vi "JSON to LVObject - Base Class - Returns Matching Type.vi"() -> ()   [LabVIEW 2017, in "Tests.lvlib" / "Type Name Handling.lvlib"]
uses:
  Weather Forecast/Weather Forecast.lvclass
  Flatten To JSON Object/Flatten To JSON Object.lvclass
  Flatten To JSON Object/Type Name Handling.ctl
  Flatten To JSON Object/Flatten To JSON Object.lvclass/Flatten To JSON Object.ctl
  Flatten To JSON Object/Write Type Name Handling.vi
  <vilib>/addons/_JKI Toolkits/Caraya/classes/Assert/Assert Equal Value and Type_Variant.vi
  Type Name Handling.lvlib
  <vilib>/addons/_JKI Toolkits/Caraya/classes/Test/Test.lvclass
  <vilib>/addons/_JKI Toolkits/Caraya/classes/Assert/Assert.lvclass
panel:
  out "error out":errorcluster
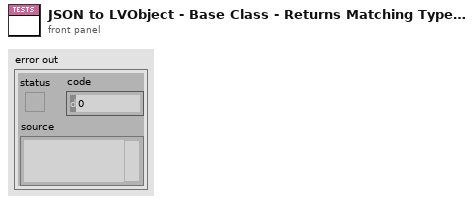
[diagram p1: front panel]
types:
  T1 = typedef "Flatten To JSON Object.lvclass/Type Name Handling.ctl" = enum16{"None", "Inline"}
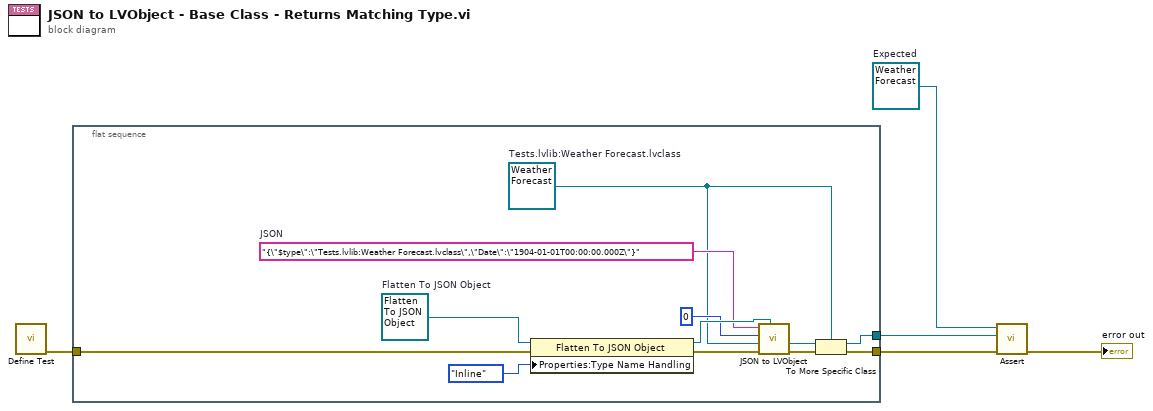
[diagram p0: block diagram]
diagram:
  w1 = refnum<class "Weather Forecast.lvclass"> refnum  # Expected
  n1 = call <vilib>:"Define Test.vi"() -> ("error out"=w5:errorcluster)  [unwired: 11 in]
  n2 = flat-sequence {
    tunnel: w5 -> [w15]
    tunnel: [w7] -> w4
    tunnel: [w9] -> w3
    frame #0 {
      w12 = "{\"$type\":\"Tests.lvlib:Weather Forecast.lvclass\",\"Date\":\"1904-01-01T00:00:00.000Z\"}"  # JSON
      w17 = refnum<class "Flatten To JSON Object.lvclass"> refnum  # Flatten To JSON Object
      w6 = refnum<class "Weather Forecast.lvclass"> refnum  # Tests.lvlib:Weather Forecast.lvclass
      n3 = property class="Flatten To JSON Object"(reference=w17, error in=w15, "Properties:Type Name Handling"=Type_Name_Handling."Inline" ("Type Name Handling")) -> (reference out=w13:refnum<class "Flatten To JSON Object.lvclass">, error out=w14:errorcluster)
      n4 = call-dynamic "JSON to LVObject.vi"("Flatten To JSON Object in"=w13, "error in (no error)"=w14, "Object Type"=w6, "Offset"=0, "JSON"=w12) -> ("error out"=w8:errorcluster, "Object"=w11:refnum<class>)  [unwired: 5 in]
      n5 = To More Specific Class(target class=w6, reference=w11, error in=w8) -> (specific class reference=w9:refnum<class "Weather Forecast.lvclass">, error out=w7:errorcluster)
    }
  }
  n6 = call-poly <vilib>:"Assert.vi"("error in (no error)"=w4, "Y"=w3, "X"=w1) -> ("error out"=→"error out":errorcluster)  [unwired: 8 in]
